vi "Read msg.vi"(8 "error in (no error)":errorcluster, 11 "Message Step in":refnum<class "Message Step.lvclass">) -> (0 "error out":errorcluster, 2 "msg":string, 3 "Message Step out":refnum<class "Message Step.lvclass">)   [LabVIEW 2017, in "Controller.lvlib" / "Message Step.lvclass"]
uses:
  Message Step.lvclass
  Message Step.lvclass/Message Step.ctl
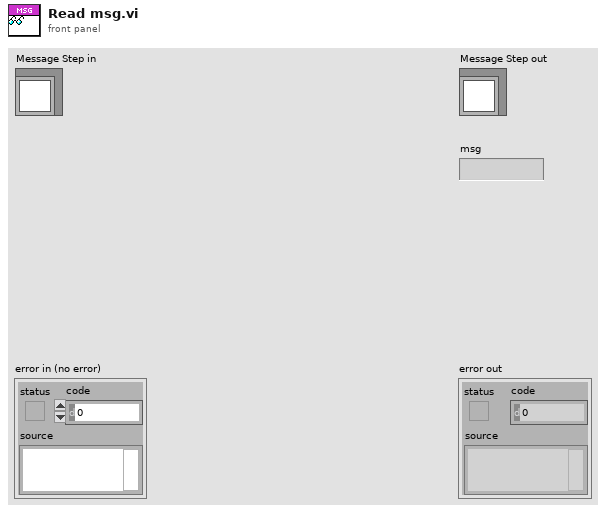
[diagram p1: front panel]
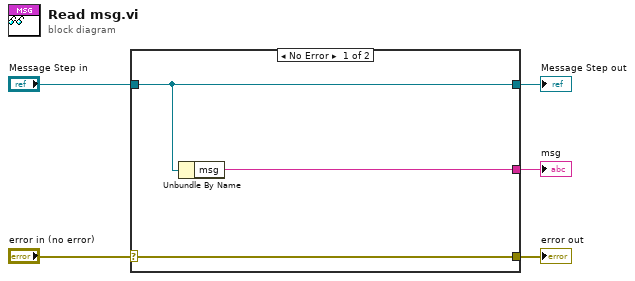
[diagram p0: block diagram]
diagram:
  n1 = case shown="No Error" "error in (no error)" {
    selector: "error in (no error)" -> [w8 w9]
    tunnel: [w8 w9] -> w4
    tunnel: [w7 w10] -> w2
    tunnel: "Message Step in" -> [w7 w10]
    tunnel: [w6 _] -> w1
    frame No Error {
      n2 = Unbundle By Name(w7) -> ("msg"=w6:string)
    }
    frame Error {
    }
  }
  "error out" <- w4
  "Message Step out" <- w2
  "msg" <- w1
